vi "testV9-PlotGraphFile.vi"() -> ()   [LabVIEW 2020]
uses:
  <vilib>/DAQmx/read.llb/DAQmx Read (Analog 2D DBL NChan NSamp).vi
  <vilib>/Analysis/baseanly.llb/Mean (DBL).vi
  <vilib>/DAQmx/miscellaneous.llb/DAQmx Fill In Error Info.vi
  <vilib>/Analysis/NI_AALBase.lvlib
  <resource>/objmgr/daqmx.rc
panel:
  out "double precision float":dbl
  out "Time Stamp":timestamp=timestamp(-21600 s since 1904-01-01)
  out "subarray 2":string[](array[string])
  out "index of element 2":i32
  out "subarray":string[](array[string])
  in  "Counter":dbl
  out ".not. (x .or. y)?":bool
  out "index of element":i32
  out "element":dbl
  out "?":timestamp
  out "Channels":refnum<k21>[](array[refnum])
  out "size(s)":i32
  out "NumDevices":u32
  out "x/y":dbl
  in  "?":T1(tab)
  out "Sampling Status":bool
  in  "Sampling Time":u32=5
  in  "Read Time (s)":u32=60
  in  "Channel List":string(combo)="Temperature"
  out "Read Count Daily":string="0" caption="Timestamp"
  out "Countdown to Read":string="0\n 6:17:48 PM" caption="Timestamp"
  out "?":string="Timestamp"
  out "?":string="File Location"
  out "Timestamp":string="7/26/2020\n 6:17:48 PM"
  in  "Play Button 2":bool
  in  "Next Button":bool
  in  "Stop Button 2":bool
  out "Graph Running":bool
  in  "Resolution":u8=10 min=10
  in  "Stop Button":bool
  in  "Play Button":bool
  out "Module 3":bool
  out "Module 2":bool
  out "Module 1":bool
  out "3":bool
  out "2":bool
  out "1":bool
  in  "Running Module":u8=1 min=1 max=3
  in  "Module 3 Task":refnum<k21>="MyTemperatureTask_2"
  out "?":waveform(dbl)(graph)
  in  "Module 3 File Data Location":path=path "E:/KMUTT/Master Degree/labviewjgsee/log/Module3"
  in  "Module 2 File Data Location":path=path "E:/KMUTT/Master Degree/labviewjgsee/log/Module2"
  in  "Module 2 Task":refnum<k21>="MyTemperatureTask_1"
  in  "Module 1 File Data Location":path=path "E:/KMUTT/Master Degree/labviewjgsee/log/Module1"
  in  "Module 1 Task":refnum<k21>="MyTemperatureTask"
  in  "DAQmx Device Name":tag="JGSEE"
  out "Table Module 1":string[][](table)
  out "Table Module 2":string[][](table)
  out "Table Module 3":string[][](table)
  in  "Select Channel Module 1":string(combo)
  out "?":string="Timestamp"
  out "Timestamp 2":string="7/26/2020\n 6:17:48 PM" caption="Timestamp"
  out "XY Graph 2":cluster{timestamp[], dbl[]}[](graph)
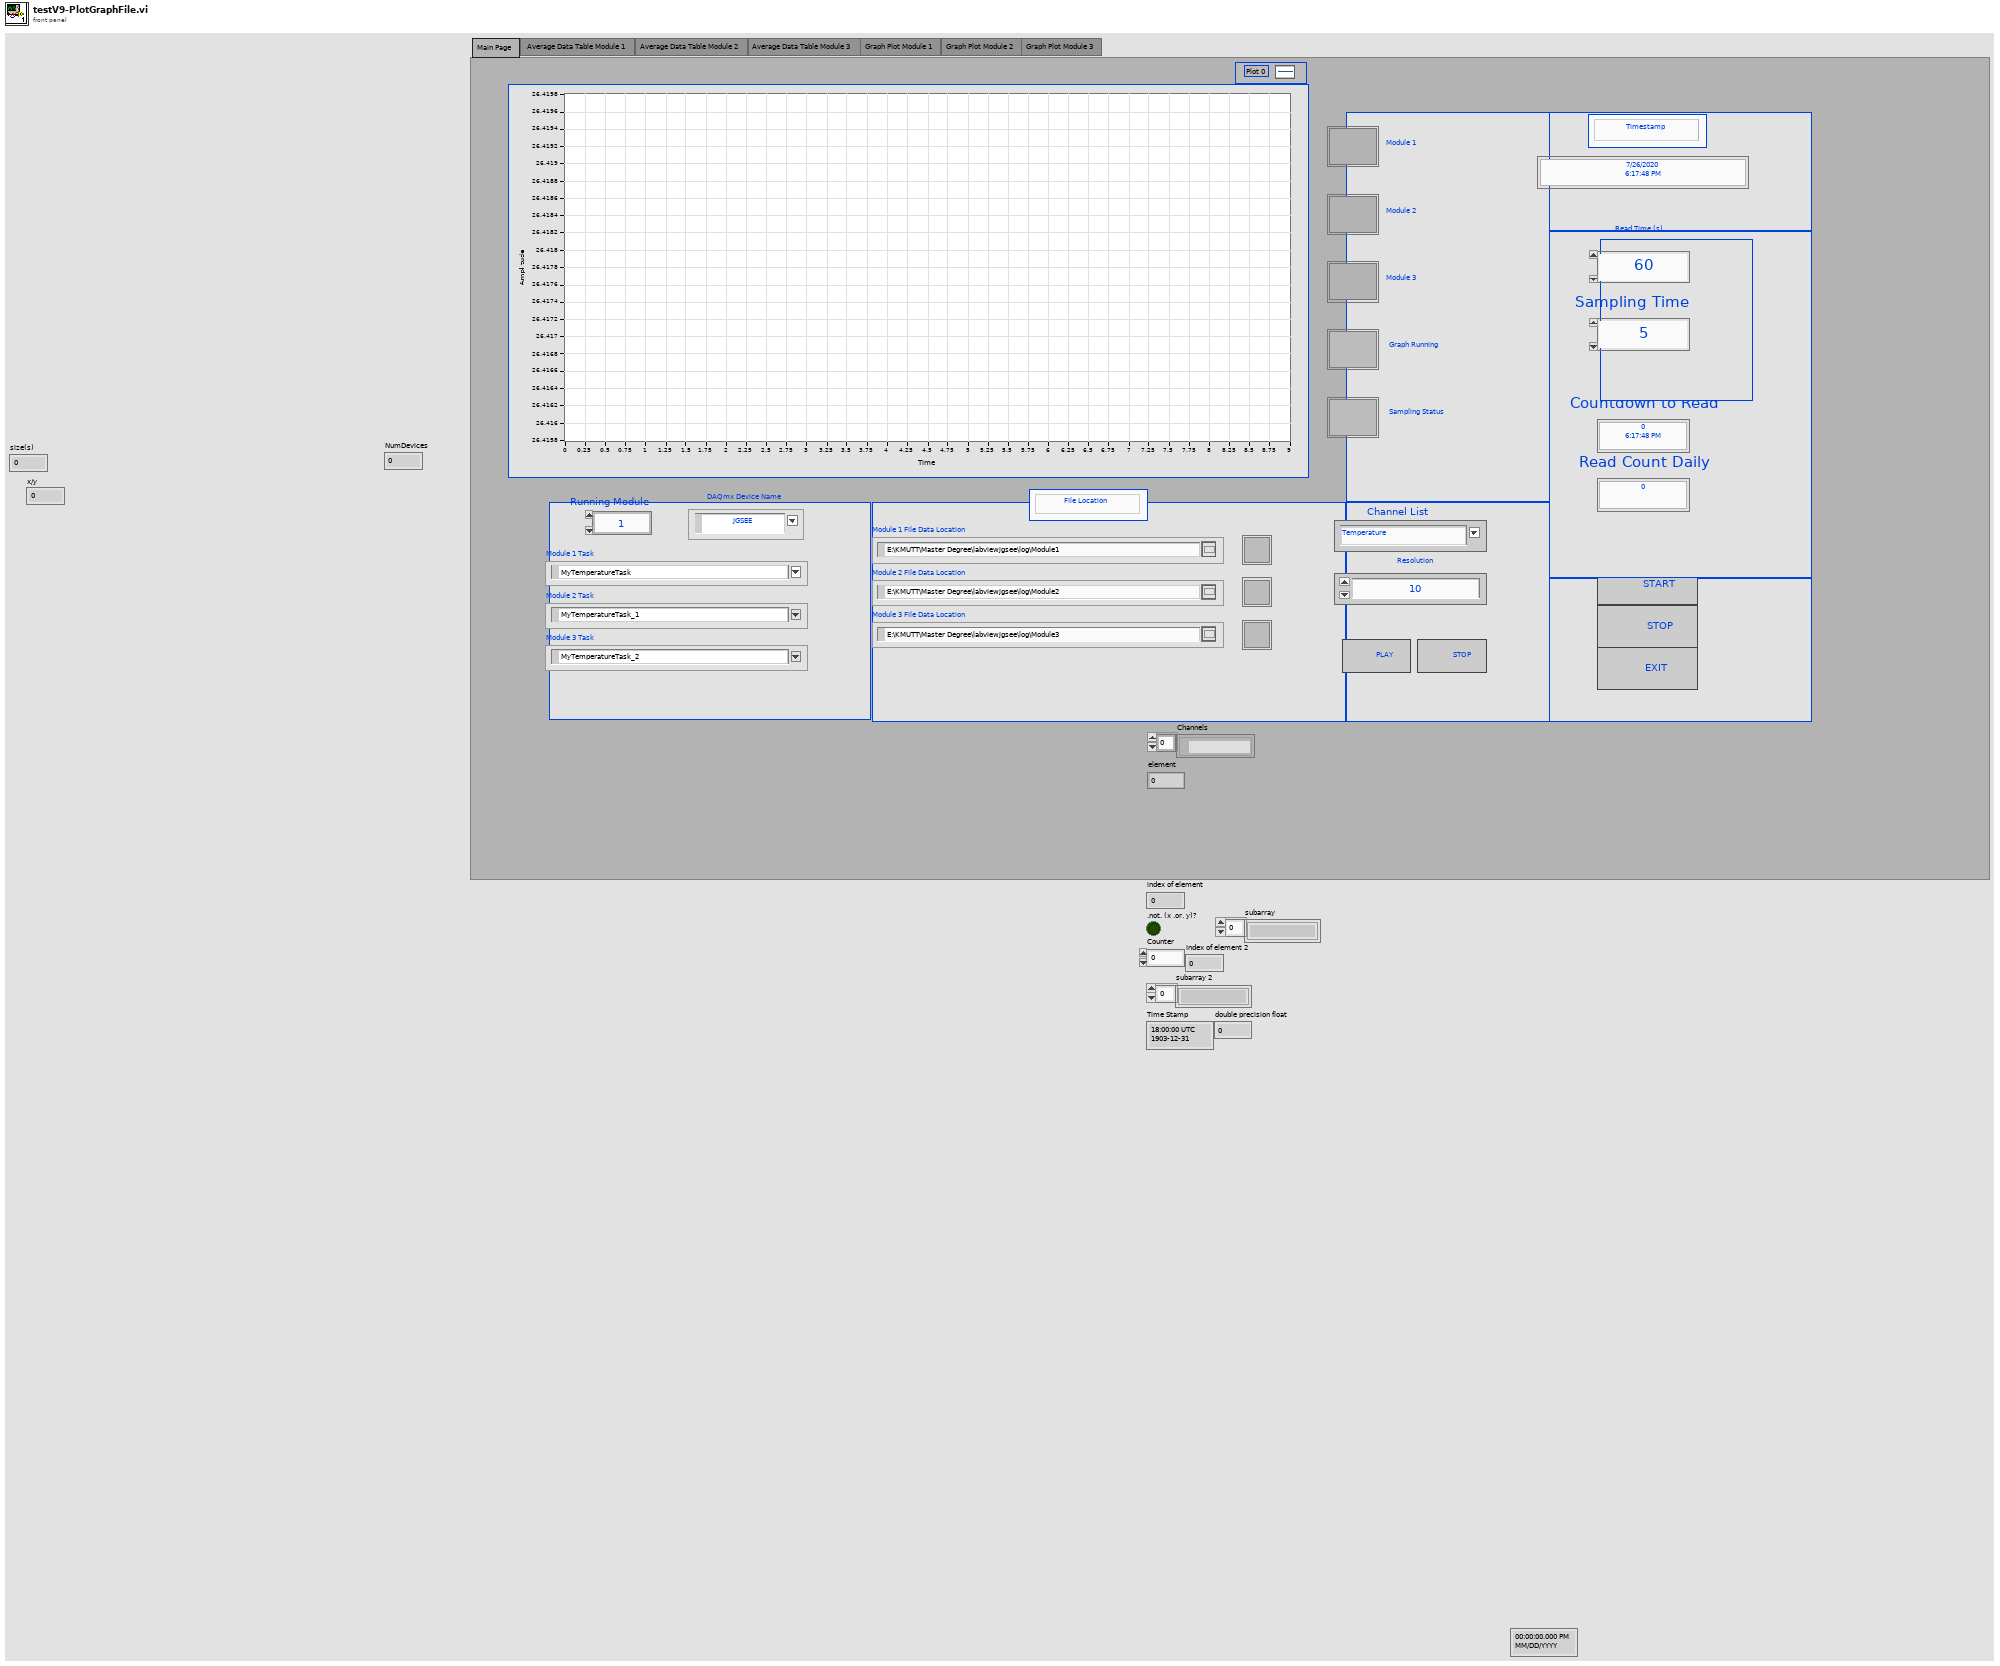
[diagram p1: front panel]
types:
  T1 = enum32{"Main Page ", " Average Data Table Module 1", "Average Data Table Module 2", "Average Data Table Module 3", "Graph Plot Module 1", "Graph Plot Module 2", "Graph Plot Module 3"}
  T2 = enum16{"open", "replace", "create", "open or create", "replace or create", "replace or create with confirmation"}
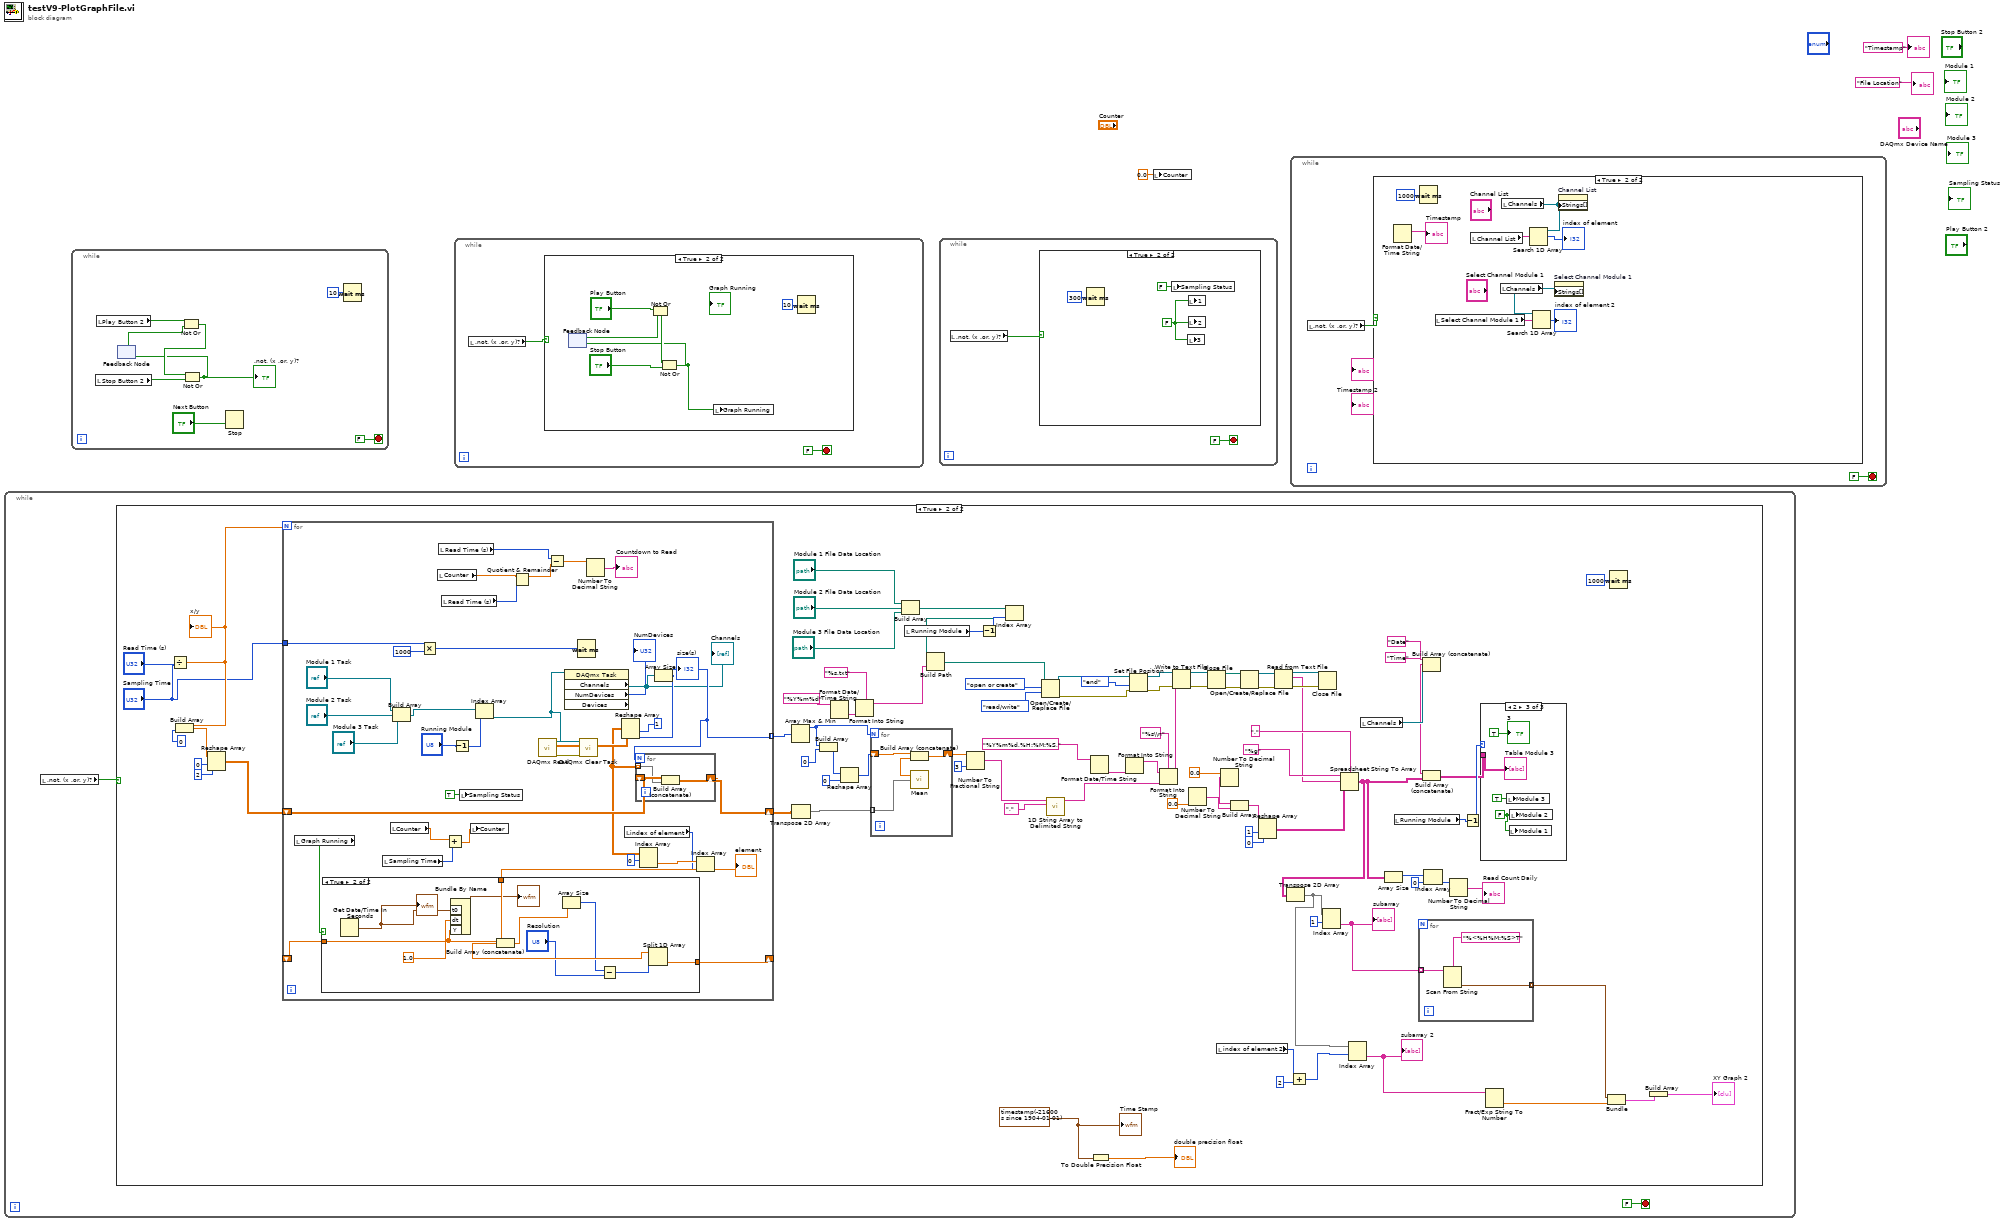
[diagram p0: block diagram]
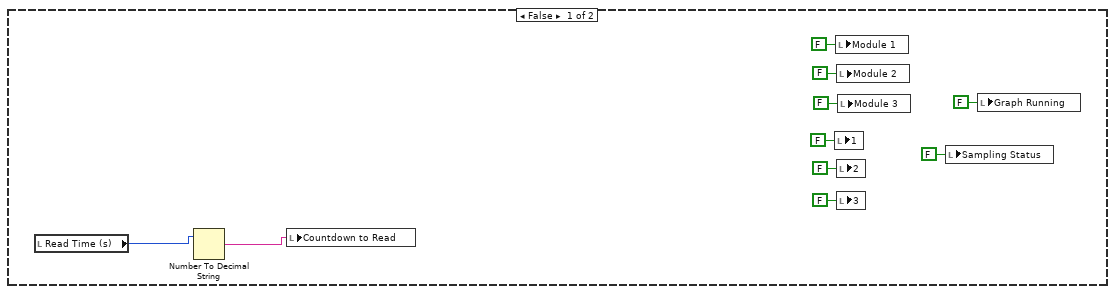
[diagram p5: hidden frame]
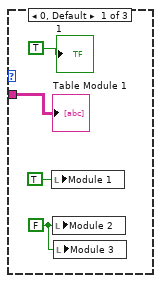
[diagram p6: hidden frame]
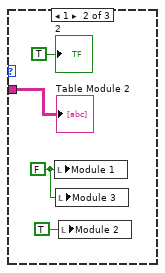
[diagram p7: hidden frame]
diagram:
  n1 = while {
    stop <- FALSE stop-if-true
    n2 = local read ".not. (x .or. y)?"() -> (w4:bool)
    n3 = case shown="True" w4 {
      frame False {
        n4 = local read "Read Time (s)"() -> (w7:u32)
        n5 = Number To Decimal String(number=w7) -> (decimal integer string=w6:string)  [unwired: 1 in]
        n6 = local write "Countdown to Read"(w6) -> ()
        n7 = local write "1"(FALSE ("1")) -> ()
        n8 = local write "Module 1"(FALSE ("Module 1")) -> ()
        n9 = local write "Module 2"(FALSE ("Module 2")) -> ()
        n10 = local write "2"(FALSE ("2")) -> ()
        n11 = local write "3"(FALSE ("3")) -> ()
        n12 = local write "Module 3"(FALSE ("Module 3")) -> ()
        n13 = local write "Sampling Status"(FALSE ("Sampling Status")) -> ()
        n14 = local write "Graph Running"(FALSE ("Graph Running")) -> ()
      }
      frame True {
        w17 = timestamp(-21600 s since 1904-01-01)
        n15 = Divide(x="Read Time (s)", y="Sampling Time") -> (x/y=w81:dbl)
        "x/y" <- w81
        n16 = Build Array(w81, 0 ("element")) -> (w85:dbl[])
        n17 = Reshape Array(w85, 0 ("dimension size"), 2 ("dimension size")) -> (w82:dbl[][])
        n18 = for {
          N: w81 -> [_]
          shift-right: [w154] -> w50
          shift-left: w82 -> [w153]
          tunnel: "Sampling Time" -> [w152]
          tunnel: [w150] -> w80 mode=indexing
          shift-right: [w134] -> _
          shift-left: _ -> [w133]
          n19 = local read "Graph Running"() -> (w132:bool)
          n20 = local read "Sampling Time"() -> (w128:u32)
          n21 = local read "Counter"() -> (w127:dbl)
          n22 = Build Array("Module 1 Task", "Module 2 Task", "Module 3 Task") -> (w145:refnum<k21>[])
          n23 = Multiply(x=w152, y=u32 1000) -> (x*y=w140:u32)
          n24 = local read "Counter"() -> (w121:dbl)
          n25 = local read "Read Time (s)"() -> (w124:u32)
          n26 = local read "Read Time (s)"() -> (w126:u32)
          n27 = Add(x=w127, y=w128) -> (x+y=w129:dbl)
          n28 = Decrement(x="Running Module") -> (x-1=w141:u8)
          n29 = local write "Sampling Status"(TRUE ("Sampling Status")) -> ()
          n30 = local write "Counter"(w129) -> ()
          n31 = Index Array(array=w145, index=w141) -> (element=w144:refnum<k21>)
          n32 = Quotient & Remainder(x=w121, y=w126) -> (x-y*floor(x/y)=w125:dbl)  [unwired: 1 out]
          n33 = call-poly <vilib>:"DAQmx Read.vi"("task/channels in"=w144) -> ("task out"=w156:refnum<k21>, "data"=w149:dbl[][], "error out"=w157:errorcluster)  [unwired: 12 in]
          n34 = Subtract(x=w124, y=w125) -> (x-y=w123:dbl)
          n35 = property class="DAQmx Task" props=["Channels", "NumDevices", "Devices"](reference=w144) -> ("Channels"=w139:refnum<k21>[], "NumDevices"=→"NumDevices":u32)  [unwired: 1 in, 3 out]
          "Channels" <- w139
          n36 = Wait (ms)(milliseconds to wait=w140) -> ()  [unwired: 1 out]
          n37 = call <vilib>:"DAQmx Clear Task.vi"("task in"=w156, "error in"=w157) -> ()  [unwired: 13 in, 1 out]
          n38 = Number To Decimal String(number=w123) -> (decimal integer string=→"Countdown to Read":string)  [unwired: 1 in]
          n39 = local read "index of element"() -> (w131:i32)
          n40 = Array Size(array=w139) -> (size(s)=w150:i32)
          "size(s)" <- w150
          n41 = Reshape Array(w149, 1 ("dimension size"), w150) -> (w138:dbl[][])
          n42 = for {
            N: w150 -> [_]
            shift-right: [w169] -> w154
            shift-left: w153 -> [w170]
            tunnel: w138 -> [w168] mode=indexing
            n43 = Build Array (concatenate)(w170, w168) -> (w169:dbl[][])
          }
          n44 = Index Array(array=w138, index (row)=0) -> (element=w136:dbl[])  [unwired: 1 in]
          n45 = Index Array(array=w136, index=w131) -> (element=w135:dbl)
          "element" <- w135
          n46 = case shown="True" w132 {
            tunnel: w135 -> [_ w165]
            tunnel: [_ w162] -> w134
            tunnel: w133 -> [_ w161]
            frame False {
            }
            frame True {
              n47 = Get Date/Time In Seconds() -> (seconds since 1Jan1904=w167:timestamp)
              "?" <- w167
              n48 = Bundle By Name("t0"=w167, "dt"=1.0, "Y"=w161) -> (→"?":waveform(dbl))  [unwired: 1 in]
              n49 = Build Array (concatenate)(w161, w165) -> (w163:dbl[])
              n50 = Array Size(array=w163) -> (size(s)=w159:i32)
              n51 = Subtract(x=w159, y="Resolution") -> (x-y=w160:i32)
              n52 = Split 1D Array(array=w163, index=w160) -> (second subarray=w162:dbl[])  [unwired: 1 out]
            }
          }
        }
        n53 = Array Max & Min(array=w80) -> (max value=w77:i32)  [unwired: 3 out]
        n54 = Transpose 2D Array(2D array=w50) -> (transposed array=w79:dbl[][])
        n55 = Build Array(w77, 0 ("element")) -> (w75:i32[])
        n56 = Format Date/Time String(time format string (%c)="%Y%m%d") -> (date/time string=w97:string)  [unwired: 2 in]
        n57 = Reshape Array(w75, 0 ("dimension size")) -> (w74:i32[])
        n58 = Format Into String(format string="%s.txt", w97) -> (resulting string=w95:string)  [unwired: 2 in, 1 out]
        n59 = for {
          N: w77 -> [_]
          tunnel: w79 -> [w174] mode=indexing
          shift-right: [w172] -> w87
          shift-left: w74 -> [w171]
          n60 = call-poly <vilib>:"Mean.vi"("X"=w174) -> ("mean"=w173:dbl)  [unwired: 1 out]
          n61 = Build Array (concatenate)(w171, w173) -> (w172:dbl[])
        }
        n62 = Build Array("Module 1 File Data Location", "Module 2 File Data Location", "Module 3 File Data Location") -> (w43:path[])
        n63 = local read "Running Module"() -> (w44:u8)
        n64 = Number To Fractional String(number=w87, precision (6)=i16 3) -> (F-format string=w88:string[])  [unwired: 2 in]
        n65 = Decrement(x=w44) -> (x-1=w42:u8)
        n66 = Index Array(array=w43, index=w42) -> (element=w41:path)
        n67 = Build Path(base path=w41, name or relative path=w95) -> (appended path=w94:path)
        n68 = Open/Create/Replace File(file path (use dialog)=w94, operation (0:open)=T2."open or create", access (0:read/write)=enum16{"read/write", "read-only", "write-only"}."read/write") -> (refnum out=w72:refnum<file>, error out=w101:errorcluster)  [unwired: 3 in, 1 out]
        n69 = call <vilib>:"1D String Array to Delimited String.vi"("delimiter"="," ("format string"), "string array"=w88) -> ("delimited string"=w93:string)  [unwired: 9 in]
        n70 = Format Date/Time String(time format string (%c)="%Y%m%d,%H:%M:%S,") -> (date/time string=w90:string)  [unwired: 2 in]
        n71 = To Double Precision Float(number=w17) -> (double precision float=→"double precision float":dbl)
        n72 = Format Into String(w90) -> (resulting string=w89:string)  [unwired: 3 in, 1 out]
        n73 = Set File Position(refnum=w72, from (0:start)=enum16{"start", "end", "current"}."end", error in=w101) -> (refnum out=w102:refnum<file>, error out=w100:errorcluster)  [unwired: 1 in]
        n74 = Format Into String(format string="%s\\n", initial string=w89, w93) -> (resulting string=w64:string)  [unwired: 1 in, 1 out]
        n75 = Write to Text File(file (use dialog)=w102, text=w64, error in=w100) -> (refnum out=w71:refnum<file>, error out=w70:errorcluster)  [unwired: 1 in, 1 out]
        n76 = Number To Decimal String(number=0.0 ("element")) -> (decimal integer string=w52:string)  [unwired: 1 in]
        n77 = Close File(refnum=w71, error in=w70) -> (path=w69:path, error out=w68:errorcluster)
        n78 = local read "index of element 2"() -> (w27:i32)
        n79 = Number To Decimal String(number=0.0 ("element")) -> (decimal integer string=w54:string)  [unwired: 1 in]
        n80 = Build Array(w54, w52) -> (w56:string[])
        n81 = Open/Create/Replace File(file path (use dialog)=w69, error in=w68) -> (refnum out=w67:refnum<file>, error out=w66:errorcluster)  [unwired: 4 in, 1 out]
        n82 = Reshape Array(w56, 1 ("dimension size"), 0 ("dimension size")) -> (w57:string[][])
        n83 = Read from Text File(file (use dialog)=w67, error in=w66) -> (refnum out=w65:refnum<file>, text=w60:string, error out=w61:errorcluster)  [unwired: 2 in, 1 out]
        n84 = Add(x=w27, y=2) -> (x+y=w24:i32)
        n85 = Close File(refnum=w65, error in=w61) -> ()  [unwired: 2 out]
        n86 = Spreadsheet String To Array(delimiter (Tab)=",", format string="%g", spreadsheet string=w60, array type (2D Dbl)=w57) -> (array=w29:string[][])
        n87 = Transpose 2D Array(2D array=w29) -> (transposed array=w25:string[][])
        n88 = Index Array(array=w25, index (row)=1 ("index")) -> (element=w23:string[])  [unwired: 1 in]
        "subarray" <- w23
        n89 = Index Array(array=w25, index (row)=w24) -> (element=w20:string[])  [unwired: 1 in]
        "subarray 2" <- w20
        n90 = local read "Channels"() -> (w35:refnum<k21>[])
        n91 = Array Size(array=w29) -> (size(s)=w33:i32[])
        n92 = local read "Running Module"() -> (w40:u8)
        n93 = for {
          tunnel: w23 -> [w107] mode=indexing
          tunnel: [w106] -> w18 mode=indexing
          n94 = Scan From String(format string="%<%H%M:%S>T", input string=w107) -> (output 1=w106:timestamp)  [unwired: 3 in, 3 out]
        }
        n95 = Build Array (concatenate)("Date", "Time", w35) -> (w34:string[])
        n96 = Build Array (concatenate)(w34, w29) -> (w38:string[][])
        n97 = Index Array(array=w33, index=0) -> (element=w31:i32)
        n98 = Number To Decimal String(number=w31) -> (decimal integer string=→"Read Count Daily":string)  [unwired: 1 in]
        n99 = Decrement(x=w40) -> (x-1=w39:u8)
        n100 = case shown="2" w39 {
          tunnel: w38 -> [w112 w116 w120]
          frame 0, Default {
            w109 = FALSE ("Module 2")
            n101 = local write "Module 1"(TRUE ("Module 1")) -> ()
            n102 = local write "Module 2"(w109) -> ()
            n103 = local write "Module 3"(w109) -> ()
            "Table Module 1" <- w112
            "1" <- TRUE ("1")
          }
          frame 1 {
            w113 = FALSE ("Module 1")
            n104 = local write "Module 1"(w113) -> ()
            n105 = local write "Module 3"(w113) -> ()
            n106 = local write "Module 2"(TRUE ("Module 2")) -> ()
            "Table Module 2" <- w116
            "2" <- TRUE ("2")
          }
          frame 2 {
            w117 = FALSE ("Module 2")
            n107 = local write "Module 3"(TRUE ("Module 3")) -> ()
            n108 = local write "Module 1"(w117) -> ()
            n109 = local write "Module 2"(w117) -> ()
            "Table Module 3" <- w120
            "3" <- TRUE ("3")
          }
        }
        n110 = Fract/Exp String To Number(string=w20) -> (number=w19:dbl[])  [unwired: 3 in, 1 out]
        n111 = Bundle(w18, w19) -> (w22:cluster{timestamp[], dbl[]})  [unwired: 1 in]
        n112 = Wait (ms)(milliseconds to wait=u32 1000) -> ()  [unwired: 1 out]
        n113 = Build Array(w22) -> (→"XY Graph 2":cluster{timestamp[], dbl[]}[])
        "Time Stamp" <- w17
      }
    }
  }
  n114 = while {
    stop <- FALSE stop-if-true
    n115 = local read "Stop Button 2"() -> (w180:bool)
    n116 = local read "Play Button 2"() -> (w181:bool)
    n117 = feedback #1() -> (w178:bool)  [unwired: 1 in]
    n118 = Not Or(1:w178, 2:w181) -> (0:w179:bool)
    n119 = Not Or(1:w180, 2:w179) -> (0:w175:bool)
    ".not. (x .or. y)?" <- w175
    n120 = feedback-in #1(w175) -> ()
    n121 = Stop(stop? (T)="Next Button") -> ()
    n122 = Wait (ms)(milliseconds to wait=u32 10) -> ()  [unwired: 1 out]
  }
  n123 = while {
    stop <- FALSE stop-if-true
    n124 = local read ".not. (x .or. y)?"() -> (w183:bool)
    n125 = case shown="True" w183 {
      frame False {
      }
      frame True {
        n126 = feedback #2() -> (w186:bool)  [unwired: 1 in]
        n127 = Not Or(1:w186, 2:"Play Button") -> (0:w187:bool)
        n128 = Not Or(1:"Stop Button", 2:w187) -> (0:w185:bool)
        n129 = feedback-in #2(w185) -> ()
        n130 = local write "Graph Running"(w185) -> ()
        n131 = Wait (ms)(milliseconds to wait=u32 10) -> ()  [unwired: 1 out]
      }
    }
  }
  n132 = while {
    stop <- FALSE stop-if-true
    n133 = local read ".not. (x .or. y)?"() -> (w191:bool)
    n134 = case shown="True" w191 {
      frame False {
      }
      frame True {
        w194 = FALSE ("1")
        n135 = Wait (ms)(milliseconds to wait=u32 300) -> ()  [unwired: 1 out]
        n136 = local write "Sampling Status"(FALSE ("Sampling Status")) -> ()
        n137 = local write "3"(w194) -> ()
        n138 = local write "1"(w194) -> ()
        n139 = local write "2"(w194) -> ()
      }
    }
  }
  n140 = local write "Counter"(0.0 ("Counter")) -> ()
  n141 = while {
    stop <- FALSE stop-if-true
    n142 = local read ".not. (x .or. y)?"() -> (w196:bool)
    n143 = case shown="True" w196 {
      frame False {
      }
      frame True {
        n144 = Format Date/Time String() -> (date/time string=→"Timestamp":string)  [unwired: 3 in]
        n145 = Wait (ms)(milliseconds to wait=u32 1000) -> ()  [unwired: 1 out]
        n146 = local read "Select Channel Module 1"() -> (w199:string)
        n147 = local read "Channel List"() -> (w203:string)
        n148 = local read "Channels"() -> (w200:refnum<k21>[])
        n149 = local read "Channels"() -> (w204:refnum<k21>[])
        n150 = Search 1D Array(1D array=w204, element=w203) -> (index of element=→"index of element":i32)  [unwired: 1 in]
        n151 = Search 1D Array(1D array=w200, element=w199) -> (index of element=→"index of element 2":i32)  [unwired: 1 in]
        n152 = property on="Select Channel Module 1" class="CmbBox"("Strings[]"=w200) -> ()  [unwired: 2 in, 2 out]
        n153 = property on="Channel List" class="CmbBox"("Strings[]"=w204) -> ()  [unwired: 2 in, 2 out]
      }
    }
  }
  "?" <- "File Location" ("String")
  "?" <- "Timestamp"
